vi "HovaCAL_Interface_GetOutputConcentration.vi"(8 "error in (no error)":errorcluster caption="Fehler (Eingang, kein Fehler)", 11 "AutoLin MFC Index":u32) -> (0 "error out":errorcluster caption="Fehler (Ausgang)", 2 "Konzentration":dbl, 3 "AutoLin MFC Index out":u32)   [LabVIEW 2020, in "Linearisierung v2.lvlib" / "Gasteiler.lvlib" / "HovaCAL_Interface.lvlib" / "Kommunikation.lvlib"]
uses:
  Kommunikation.lvlib
  Aktion_FGV_HovaCAL_Interface_GetData.ctl
  Aktion_FGV_HovaCAL_Interface_SetData.ctl
  Controls/Pump Concentration Mode.ctl
  Controls/Controls.lvlib
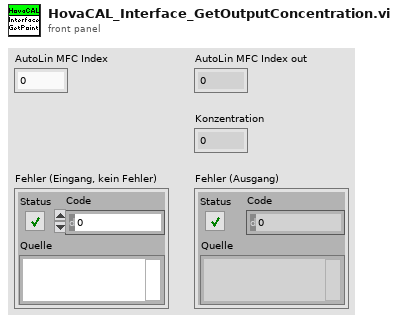
[diagram p1: front panel]
types:
  T1 = typedef "Linearisierung v2.lvlib/Gasteiler.lvlib/HovaCAL_Interface.lvlib/Kommunikation.lvlib/Aktion_FGV_HovaCAL_Interface_GetData.ctl" = enum16{"lesen", "SystemInfo", "MFC Info", "actual Values", "Limits", "first contact", "reset after read"}
  T2 = typedef "Linearisierung v2.lvlib/Gasteiler.lvlib/HovaCAL_Interface.lvlib/Controls.lvlib/Info Cluster.ctl" = cluster{"device":string, "version":string, "number of mfc":i32, "number of pumps":i32, "number of temp controllers":i32, "number of mfs":i32, "number of balances":i32}
  T3 = typedef "Linearisierung v2.lvlib/Gasteiler.lvlib/HovaCAL_Interface.lvlib/Kommunikation.lvlib/Aktion_FGV_HovaCAL_Interface_SetData.ctl" = enum16{"lesen", "Konzentrationen", "Pumpen Parameter", "Pumpe Konzentration", "Pumpe run", "Temperaturen", "Fluss", "Limits", "init"}
  T4 = typedef "Linearisierung v2.lvlib/Gasteiler.lvlib/HovaCAL_Interface.lvlib/Controls.lvlib/Pump Dry Mode.ctl" = i32
  T5 = typedef "Linearisierung v2.lvlib/Gasteiler.lvlib/HovaCAL_Interface.lvlib/Controls.lvlib/Pump Control Mode.ctl" = u32
  T6 = typedef "Linearisierung v2.lvlib/Gasteiler.lvlib/HovaCAL_Interface.lvlib/Controls.lvlib/Pump Concentration Mode.ctl" = i32
  T7 = typedef "Linearisierung v2.lvlib/Gasteiler.lvlib/HovaCAL_Interface.lvlib/Controls.lvlib/Reagent.ctl" = i32
  T8 = cluster{"Input Concentrations (Ausgang)":cluster{"input concentration setpoint":dbl, "output concentration setpoint":dbl, "output concentration":dbl, "output concentration dry":dbl}[], "Cluster":cluster{"Temp Cluster":cluster{"temp SP":dbl, "temp":dbl, "humidity":dbl}[], "PumpModeGeneral-Cluster":cluster{"running?":bool, "dry mode":T4, "control mode":T5}, "PumpMode-Cluster":cluster{"Speed":dbl, "concentratio mode":T6, "Reagent":T7, "Molarity":dbl, "density":dbl, "syringe":dbl, "pumpe_a":dbl}[], "Pump Concentrations-Cluster":cluster{"reagent conc SP":dbl, "reagent conc":dbl, "reagent conc dry":dbl, "water conc SP":dbl, "water conc":dbl, "water conc dry":dbl}[], "Flow Output Cluster (Ausgang)":cluster{"total flow setpoint":dbl, "total flow":dbl}, "Pump MassFlow-Cluster":cluster{"reagent mf SP":dbl, "reagent mf":dbl, "water mf SP":dbl, "water mf":dbl, "water/reagent mf SP":dbl, "water/reagent mf":dbl}[], "MFC Flows-Cluster":cluster{"MFC  actual flow l/min":dbl, "MFC expected flow l/min":dbl}[]}}
  T9 = cluster{"input concentration setpoint":dbl, "output concentration setpoint":dbl, "output concentration":dbl, "output concentration dry":dbl}[]
  T10 = cluster{"input concentration setpoint":dbl, "output concentration setpoint":dbl, "output concentration":dbl, "output concentration dry":dbl}
  T11 = cluster{"input concentration setpoint":dbl, "output concentration setpoint":dbl}[]
  T12 = cluster{"input concentration setpoint":dbl, "output concentration setpoint":dbl}
  T13 = cluster{"concentratio mode":T6, "Reagent":T7, "Molarity":dbl, "density":dbl, "syringe":dbl, "pump_a":dbl}[]
  T14 = typedef "Linearisierung v2.lvlib/Gasteiler.lvlib/HovaCAL_Interface.lvlib/Controls.lvlib/Pump Concentration.ctl" = cluster{"reagent conc SP":dbl, "water conc SP":dbl}
  T15 = cluster{"reagent conc SP":dbl, "reagent conc":dbl, "reagent conc dry":dbl, "water conc SP":dbl, "water conc":dbl, "water conc dry":dbl}[]
  T16 = cluster{"concentratio mode":T6, "Reagent":T7, "Molarity":dbl, "density":dbl, "syringe":dbl, "pump_a":dbl}
  T17 = cluster{"reagent conc SP":dbl, "reagent conc":dbl, "reagent conc dry":dbl, "water conc SP":dbl, "water conc":dbl, "water conc dry":dbl}
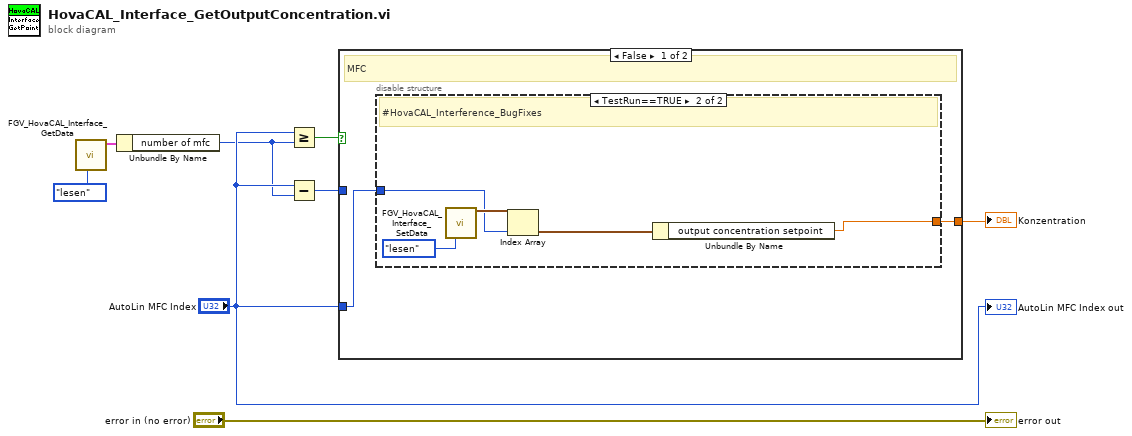
[diagram p0: block diagram]
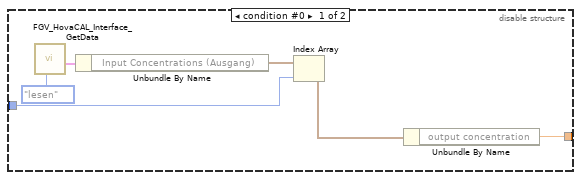
[diagram p2: hidden frame]
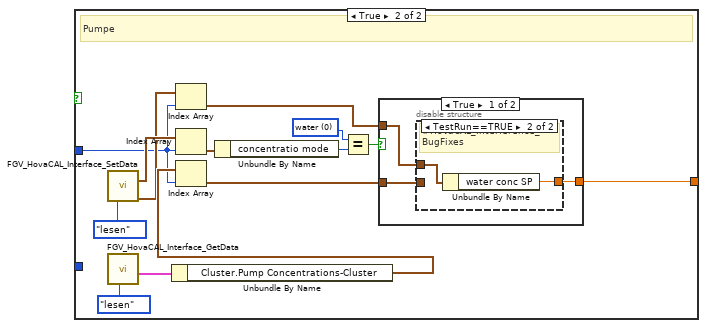
[diagram p3: hidden frame]
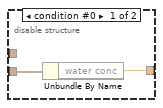
[diagram p4: hidden frame]
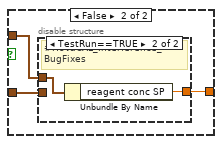
[diagram p5: hidden frame]
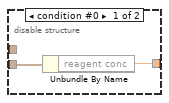
[diagram p6: hidden frame]
diagram:
  n1 = call "FGV_HovaCAL_Interface_GetData.vi"("Aktion"=Aktion_FGV_HovaCAL_Interface_GetData."lesen") -> ("System Cluster out"=w7:T2)  [unwired: 6 in, 4 out]
  n2 = Unbundle By Name(w7) -> ("number of mfc"=w5:i32)
  n3 = Greater Or Equal?(x="AutoLin MFC Index", y=w5) -> (x >= y?=w4:bool)
  n4 = Subtract(x="AutoLin MFC Index", y=w5) -> (x-y=w3:u32)
  n5 = case shown="False" w4 {
    tunnel: "AutoLin MFC Index" -> [w9 _]
    tunnel: w3 -> [_ w22]
    tunnel: [w10 w28] -> w1
    frame False {
      # "MFC"
      n6 = disable-structure shown="TestRun==TRUE" {
        disable-tunnel: [w16 w21] -> w10
        disable-tunnel: w9 -> [w11 w18]
        frame condition #0 {
          n7 = call "FGV_HovaCAL_Interface_GetData.vi"("Aktion"=Aktion_FGV_HovaCAL_Interface_GetData."lesen") -> ("actual Values Cluster out"=w15:T8)  [unwired: 6 in, 4 out]
          n8 = Unbundle By Name(w15) -> ("Input Concentrations (Ausgang)"=w12:T9)
          n9 = Index Array(array=w12, index=w11) -> (element=w13:T10)
          n10 = Unbundle By Name(w13) -> ("output concentration"=w16:dbl)
        }
        frame condition #1 (active) {
          # "#HovaCAL_Interference_BugFixes"
          n11 = call "FGV_HovaCAL_Interface_SetData.vi"("Aktion"=Aktion_FGV_HovaCAL_Interface_SetData."lesen") -> ("Set Values Cluster out"=w20:T11)  [unwired: 8 in, 6 out]
          n12 = Index Array(array=w20, index=w18) -> (element=w19:T12)
          n13 = Unbundle By Name(w19) -> ("output concentration setpoint"=w21:dbl)
        }
      }
    }
    frame True {
      w32 = T6 0 items=["water", "reagent"] ("x")
      # "Pumpe"
      n14 = call "FGV_HovaCAL_Interface_SetData.vi"("Aktion"=Aktion_FGV_HovaCAL_Interface_SetData."lesen") -> ("PumpMode-Cluster out"=w30:T13, "Pump Concentrations-Cluster out"=w24:T14[])  [unwired: 8 in, 5 out]
      n15 = call "FGV_HovaCAL_Interface_GetData.vi"("Aktion"=Aktion_FGV_HovaCAL_Interface_GetData."lesen") -> ("actual Values Cluster out"=w26:T8)  [unwired: 6 in, 4 out]
      n16 = Unbundle By Name(w26) -> ("Cluster.Pump Concentrations-Cluster"=w25:T15)
      n17 = Index Array(array=w24, index=w22) -> (element=w23:T14)
      n18 = Index Array(array=w30, index=w22) -> (element=w34:T16)
      n19 = Index Array(array=w25, index=w22) -> (element=w29:T17)
      n20 = Unbundle By Name(w34) -> ("concentratio mode"=w33:T6)
      n21 = Equal?(x=w32, y=w33) -> (x = y?=w31:bool)
      n22 = case shown="True" w31 {
        tunnel: [w38 w45] -> w28
        tunnel: w29 -> [w37 w44]
        tunnel: w23 -> [w36 w43]
        frame True {
          n23 = disable-structure shown="TestRun==TRUE" {
            disable-tunnel: [w40 w42] -> w38
            disable-tunnel: w37 -> [w39 _]
            disable-tunnel: w36 -> [_ w41]
            frame condition #0 {
              n24 = Unbundle By Name(w39) -> ("water conc"=w40:dbl)
            }
            frame condition #1 (active) {
              # "#HovaCAL_Interference_BugFixes"
              n25 = Unbundle By Name(w41) -> ("water conc SP"=w42:dbl)
            }
          }
        }
        frame False {
          n26 = disable-structure shown="TestRun==TRUE" {
            disable-tunnel: [w47 w49] -> w45
            disable-tunnel: w44 -> [w46 _]
            disable-tunnel: w43 -> [_ w48]
            frame condition #0 {
              n27 = Unbundle By Name(w46) -> ("reagent conc"=w47:dbl)
            }
            frame condition #1 (active) {
              # "#HovaCAL_Interference_BugFixes"
              n28 = Unbundle By Name(w48) -> ("reagent conc SP"=w49:dbl)
            }
          }
        }
      }
    }
  }
  "Konzentration" <- w1
  "error out" <- "error in (no error)"
  "AutoLin MFC Index out" <- "AutoLin MFC Index"
